vi "SaveDataToDiskAsGlimpse_openonce.vi"(0 "refnum in":refnum<file>, 1 "Array (U8)":u8[][](array[numeric]), 3 "Data type":enum16{"U8", "U16"}(ring), 4 "Array (I16)":i16[][](array[numeric]), 5 "error in":errorcluster) -> (6 "refnum out":refnum<file>, 8 "error out":errorcluster)   [LabVIEW 2014]
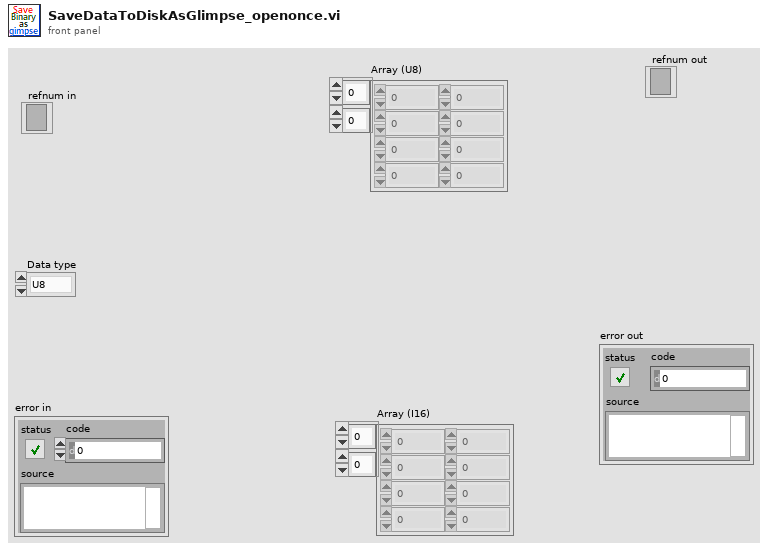
[diagram p1: front panel]
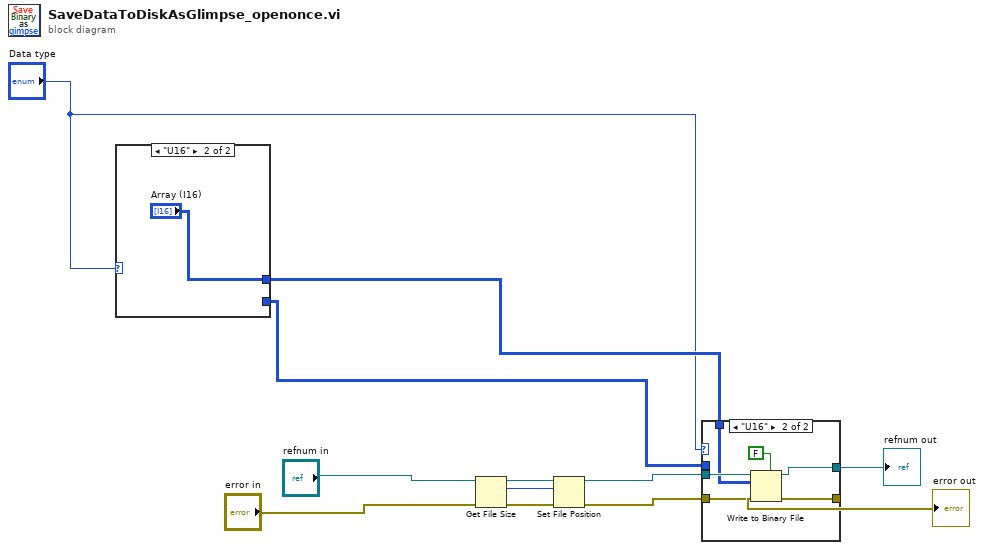
[diagram p0: block diagram]
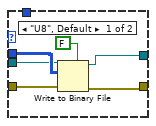
[diagram p2: hidden frame]
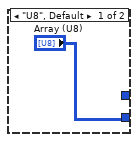
[diagram p3: hidden frame]
diagram:
  n1 = case shown="\"U16\"" "Data type" {
    tunnel: [_ "Array (I16)"] -> w9
    tunnel: ["Array (U8)" _] -> w7
    frame "U8", Default {
    }
    frame "U16" {
    }
  }
  n2 = Get File Size(file="refnum in", error in="error in") -> (refnum out=w6:refnum<file>, size (in bytes)=w5:i64, 0:w4:errorcluster)
  n3 = Set File Position(offset (in bytes) (0)=w5, refnum=w6, error in=w4) -> (refnum out=w12:refnum<file>, error out=w11:errorcluster)  [unwired: 1 in]
  n4 = case shown="\"U16\"" "Data type" {
    tunnel: w12 -> [w16 w25]
    tunnel: w11 -> [w18 w24]
    tunnel: [w17 w23] -> w10
    tunnel: w9 -> [_ w22]
    tunnel: w7 -> [w19 _]
    tunnel: [w15 w21] -> w2
    frame "U8", Default {
      n5 = Write to Binary File(file (use dialog)=w16, data=w19, error in=w18, 5:FALSE ("prepend array or string size? (T)")) -> (refnum out=w15:refnum<file>, error out=w17:errorcluster)  [unwired: 2 in, 1 out]
    }
    frame "U16" {
      n6 = Write to Binary File(file (use dialog)=w25, data=w22, error in=w24, 5:FALSE ("prepend array or string size? (T)")) -> (refnum out=w21:refnum<file>, error out=w23:errorcluster)  [unwired: 2 in, 1 out]
    }
  }
  "error out" <- w10
  "refnum out" <- w2
